vi "Log Configuration.vi"(8 "error in (no error)":errorcluster, 11 "Sift Stream in":refnum<class "Sift Stream.lvclass">) -> (0 "error out":errorcluster, 3 "Sift Stream out":refnum<class "Sift Stream.lvclass">)   [LabVIEW 2024, in "Sift Stream.lvlib" / "Sift Stream.lvclass"]
uses:
  Sift Stream.lvclass
  Sift Stream.lvclass/Sift Stream.ctl
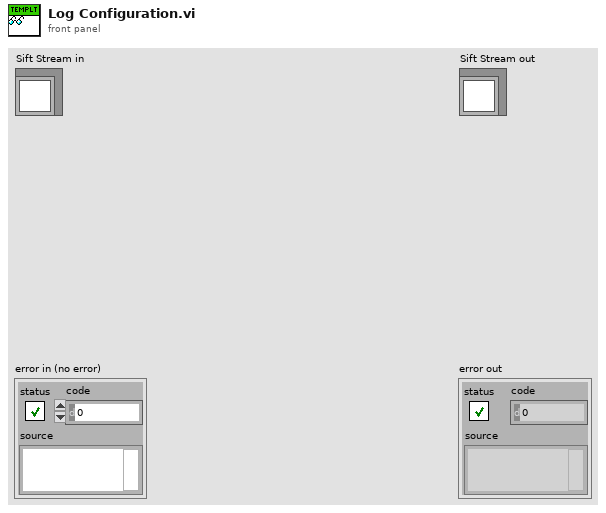
[diagram p1: front panel]
types:
  T1 = typedef "Sift Stream.lvlib/Sift Stream.lvclass/Sift Stream Parameters.ctl" = cluster{"API gRPC URL":string, "API REST URL":string, "API Key":string, "Asset Name":string, "Data Rate":dbl, "Stream Names":string[], "Sift Client":refnum<class "Sift Client.lvclass">, "Session Error":errorcluster, "Stop Notifier":refnum<notifier>, "Channel Name Prefix":string}
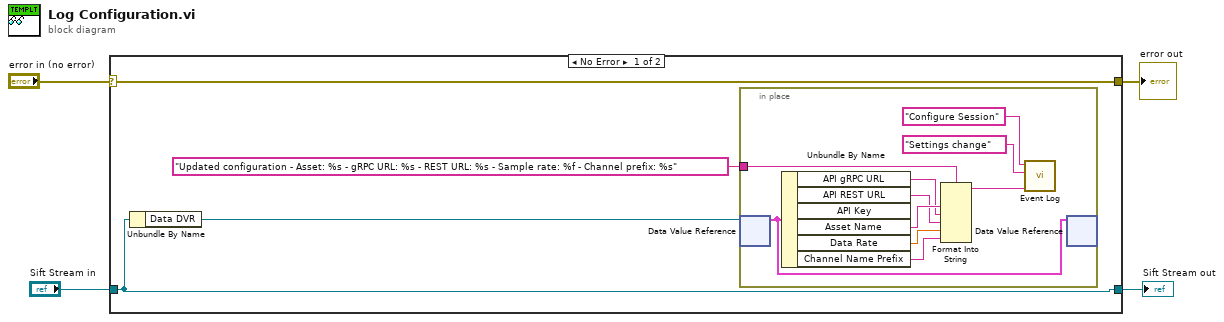
[diagram p0: block diagram]
diagram:
  n1 = case shown="No Error" "error in (no error)" {
    selector: "error in (no error)" -> [w8 w19]
    tunnel: [w8 w19] -> w3
    tunnel: [w7 w20] -> w1
    tunnel: "Sift Stream in" -> [w7 w20]
    frame No Error {
      n2 = Unbundle By Name(w7) -> ("Data DVR"=w6:refnum<data-value>)
      n3 = in-place {
        in-place-border: "Updated configuration - Asset: %s - gRPC URL: %s - REST URL: %s - Sample rate: %f - Channel prefix: %s" -> [w18]
        n4 = in-place-dvr #1(w6) -> (w9:T1)  [unwired: 1 out]
        n5 = Unbundle By Name(w9) -> ("API gRPC URL"=w13:string, "API REST URL"=w12:string, "Asset Name"=w14:string, "Data Rate"=w11:dbl, "Channel Name Prefix"=w10:string)  [unwired: 1 out]
        n6 = Format Into String(format string=w18, w14, w13, w12, w11, w10) -> (resulting string=w15:string)  [unwired: 2 in, 1 out]
        n7 = call "Event Log.vi"("Message"=w15, "Event Type"="Settings change", "Location"="Configure Session") -> ()  [unwired: 9 in]
        n8 = in-place-dvr #1(w9) -> ()  [unwired: 2 out]
      }
    }
    frame Error {
    }
  }
  "error out" <- w3
  "Sift Stream out" <- w1
